vi "Scan List.vi"(8 "error in (no error)":errorcluster, 10 "通道数":i32, 11 "VISA resource name":refnum<visa-resource-name>) -> (0 "error out":errorcluster, 3 "VISA resource name out":refnum<visa-resource-name>)   [LabVIEW 2015]
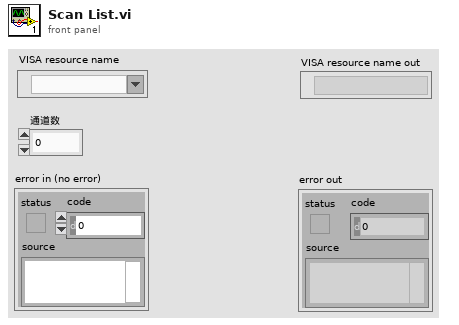
[diagram p1: front panel]
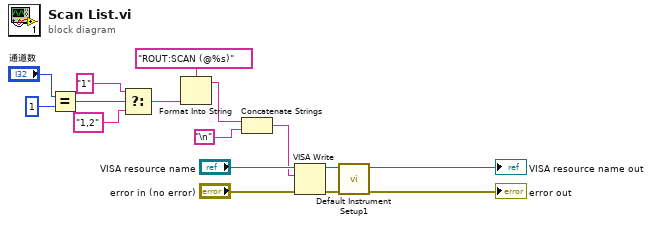
[diagram p0: block diagram]
diagram:
  n1 = Equal?(x="通道数", y=1) -> (x = y?=w4:bool)
  n2 = Select(t="1" ("Reset Command"), s=w4, f="1,2" ("Reset Command")) -> (s? t:f=w2:string)
  n3 = Format Into String(format string="ROUT:SCAN (@%s)" ("Reset Command"), w2) -> (resulting string=w9:string)  [unwired: 2 in, 1 out]
  n4 = Concatenate Strings(w9, "\n") -> (w11:string)
  n5 = VISA Write(VISA resource name="VISA resource name", write buffer=w11, error in (no error)="error in (no error)") -> (VISA resource name out=w14:refnum<visa-resource-name>, error out=w13:errorcluster)  [unwired: 1 out]
  n6 = call "Default Instrument Setup1.vi"("error in (no error)"=w13, "VISA resource name"=w14) -> ("error out"=→"error out":errorcluster, "VISA resource name out"=→"VISA resource name out":refnum<visa-resource-name>)  [unwired: 8 in]
